vi "Test Handle Suite Result.vi"(8 "error in (no error)":errorcluster, 11 "Result Model Result Recording Test in":refnum<class "Result Model Result Recording Test.lvclass">) -> (0 "error out":errorcluster, 3 "Result Model Result Recording Test out":refnum<class "Result Model Result Recording Test.lvclass">)   [LabVIEW 2020, in "Result Model Result Recording Test.lvclass"]
uses:
  Result Model Result Recording Test.lvclass
  source/Core/Result/Type.ctl
  source/Core/Result/Result.lvlib
  source/Core/Result/Status.ctl
  source/Core/Result/Result.ctl
  source/User Interface/Result Model/Result Model.lvclass
  ae2c71b8-32bb-49d1-8500-0119bfec74ff.vi
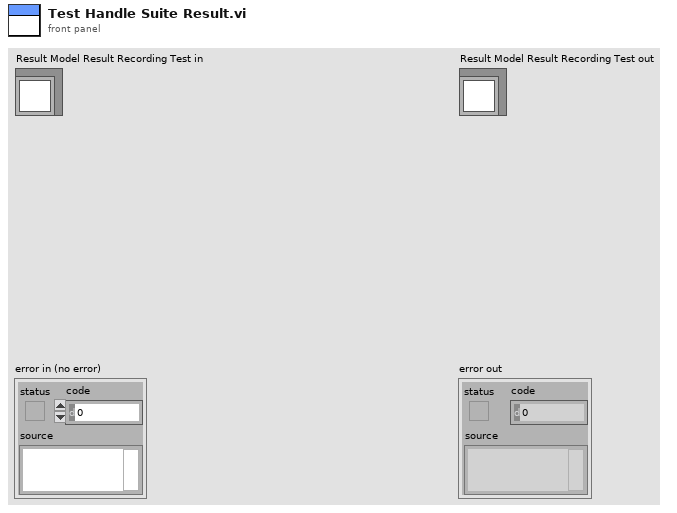
[diagram p1: front panel]
types:
  T1 = typedef "Result.lvlib/Result.ctl" = cluster{"Name":string, "Description":string, "Status":T2, "Result Type":T3, "Execution Time":dbl, "Data":cluster{"Expected":variant, "Actual":variant, "Delta":variant}}
  T2 = typedef "Result.lvlib/Status.ctl" = enum16{"", "Passed", "Failed", "Error", "Skipped", "Setup Error", "Broken", "Teardown Error"}
  T3 = typedef "Result.lvlib/Type.ctl" = enum16{"Test Case", "Test Suite", "Test Run", "Pass", "Fail", "Skip", "Pass if", "Fail if", "Pass if Error", "Fail if Error", "Pass if Equal", "Fail if Equal"}
  T4 = cluster{"Left Cell String":string, "Child Text":string[], "Child Tag":string, "Item Indent":i32, "Child Only?":bool, "Glyph Index":i32}[]
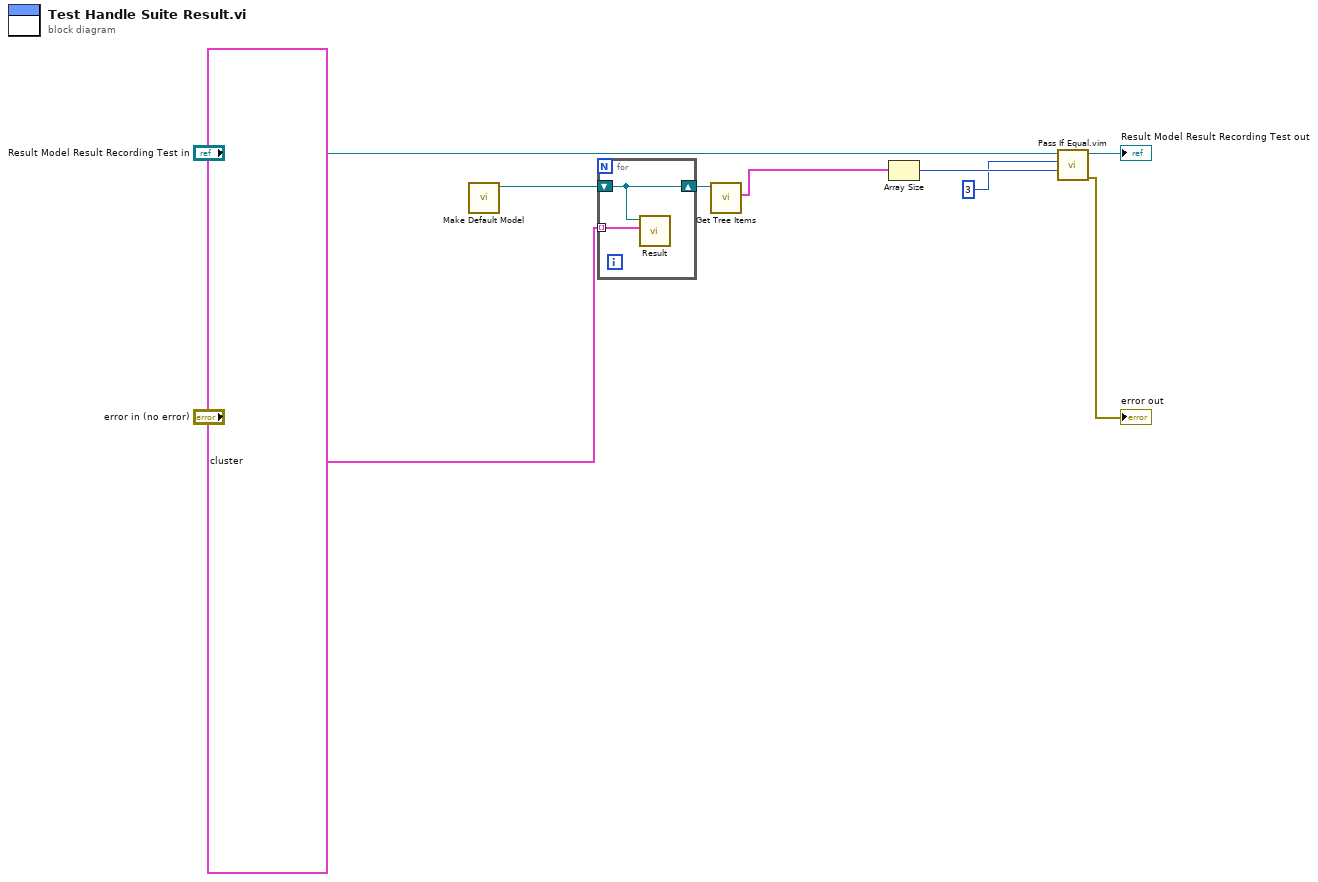
[diagram p0: block diagram]
diagram:
  n1 = call "Make Default Model.vi"() -> ("Result Model out"=w9:refnum<class "Result Model.lvclass">)  [unwired: 10 in, 1 out]
  n2 = for {
    tunnel: T1[] [{"Name"="Case.lvclass:Test Method.vi", "Description"="Failed:\nMessage", "Status"=enum."Failed", "Result Type"=enum."Test Case", "Execution Time"=0.107, "Data"={"Expected"=variant, "Actual"=variant, "Delta"=variant}}, {"Name"="Case.lvclass:Test Method2.vi", "Description"="", "Status"=enum."Passed", "Result Type"=enum."Test Case", "Execution Time"=0.0, "Data"={"Expected"=variant, "Actual"=variant, "Delta"=variant}}, {"Name"="Case.lvclass", "Description"="", "Status"=enum."Failed", "Result Type"=enum."Test Suite", "Execution Time"=0.0, "Data"={"Expected"=variant, "Actual"=variant, "Delta"=variant}}, {"Name"="Suite Name", "Description"="", "Status"=enum."Passed", "Result Type"=enum."Test Run", "Execution Time"=0.0, "Data"={"Expected"=variant, "Actual"=variant, "Delta"=variant}}] ("Results") -> [w11] mode=indexing
    shift-right: [w10] -> w7
    shift-left: w9 -> [w10]
    n3 = call-dynamic "Result.vi"("Results"=w11, "Result Model by Reference In"=w10) -> ()  [unwired: 9 in, 1 out]
  }
  n4 = call "Get Tree Items.vi"("Result Model by Reference In"=w7) -> ("Tree Items"=w6:T4)  [unwired: 9 in, 1 out]
  n5 = Array Size(array=w6) -> (size(s)=w2:i32)
  n6 = call "Pass If Equal.vim"("Actual"=w2, "Expected"=3 ("size(s)"), "LUnit Test Case In"="Result Model Result Recording Test in") -> ("error out"=→"error out":errorcluster, "LUnit Test Case Out"=→"Result Model Result Recording Test out":refnum<class "Result Model Result Recording Test.lvclass">)  [unwired: 7 in]
